vi "RSZVB Write From File To Instrument.vi"(8 "error in (no error)":errorcluster {"code" format="%.0x"}, 9 "Destination":path=path "D:/user/data/test.hcp", 10 "Source":path=path "C:/test.hcp", 11 "VISA session":refnum<visa-resource-name>) -> (0 "error out":errorcluster {"code" format="%.0x"}, 3 "dup VISA session":refnum<visa-resource-name>)   [LabVIEW 2011]
doc: "This VI is used to read data from the host computer and write it to a user specified file in the instrument.\n\nRemote-control command(s):\nSYSTem:COMMunicate:GPIB[:SELF]:RTERminator LFEOI | EOI\nMMEMory:DATA '<file_name>', <data>"
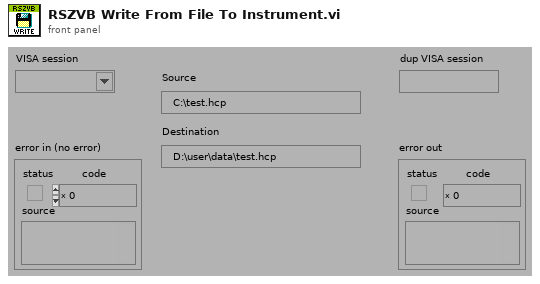
[diagram p1: front panel]
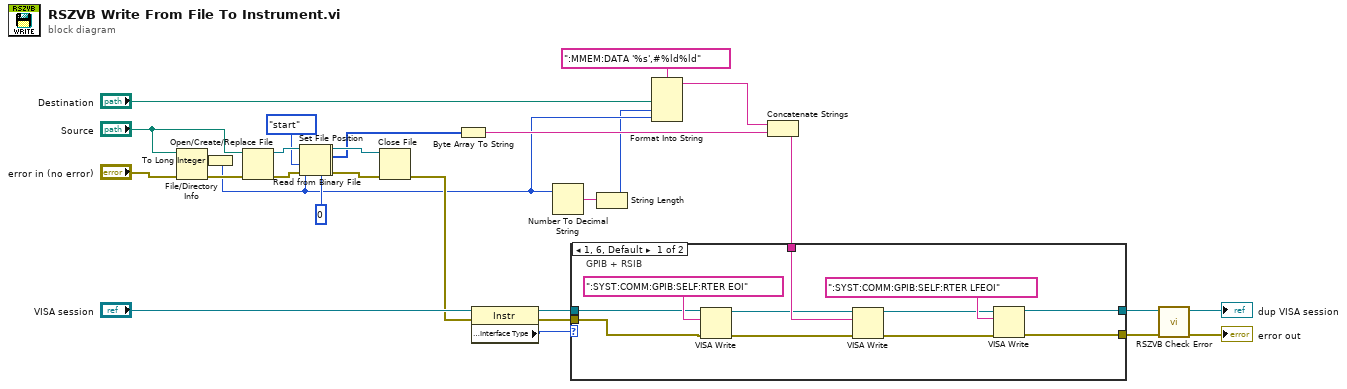
[diagram p0: block diagram]
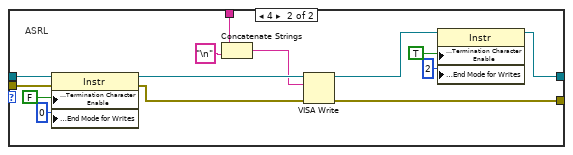
[diagram p2: hidden frame]
diagram:
  n1 = File/Directory Info(path="Source", error in="error in (no error)") -> (size=w3:i64, error out=w19:errorcluster)  [unwired: 5 out]
  n2 = To Long Integer(number=w3) -> (32bit integer=w9:i32)
  n3 = Open/Create/Replace File(file path (use dialog)="Source", error in=w19) -> (refnum out=w17:refnum<file>, error out=w21:errorcluster)  [unwired: 4 in, 1 out]
  n4 = Set File Position(refnum=w17, from (0:start)=enum16{"start", "end", "current"}."start" ("pos mode (0:2)"), error in=w21) -> (refnum out=w2:refnum<file>, error out=w1:errorcluster)  [unwired: 1 in]
  n5 = Read from Binary File(5:u8 0 ("byte stream type"), 8:w1, 10:w9, 11:w2) -> (0:w20:errorcluster, 2:w13:u8[], 3:w18:refnum<file>)  [unwired: 2 in, 1 out]
  n6 = Close File(refnum=w18, error in=w20) -> (error out=w11:errorcluster)  [unwired: 1 out]
  n7 = Byte Array To String(unsigned byte array=w13) -> (string=w12:string)
  n8 = property class="Instr"(reference="VISA session", error in=w11) -> (reference out=w27:refnum<visa-resource-name>, error out=w26:errorcluster, "Interface Information:Interface Type"=w25:u16)
  n9 = Number To Decimal String(number=w9) -> (decimal integer string=w10:string)  [unwired: 1 in]
  n10 = String Length(string=w10) -> (length=w8:i32)
  n11 = Format Into String(format string=":MMEM:DATA '%s',#%ld%ld", "Destination", w8, w9) -> (resulting string=w30:string)  [unwired: 2 in, 1 out]
  n12 = Concatenate Strings(w30, w12) -> (w28:string)
  n13 = case shown="1, 6, Default" w25 {
    tunnel: [w41 w45] -> w4
    tunnel: [w40 w44] -> w5
    tunnel: w28 -> [w39 w49]
    tunnel: w27 -> [w32 w55]
    tunnel: w26 -> [w31 w54]
    frame 1, 6, Default {
      # "GPIB + RSIB"
      n14 = VISA Write(VISA resource name=w32, write buffer=":SYST:COMM:GPIB:SELF:RTER EOI", error in (no error)=w31) -> (VISA resource name out=w36:refnum<visa-resource-name>, error out=w33:errorcluster)  [unwired: 1 out]
      n15 = VISA Write(VISA resource name=w36, write buffer=w39, error in (no error)=w33) -> (VISA resource name out=w35:refnum<visa-resource-name>, error out=w34:errorcluster)  [unwired: 1 out]
      n16 = VISA Write(VISA resource name=w35, write buffer=":SYST:COMM:GPIB:SELF:RTER LFEOI", error in (no error)=w34) -> (VISA resource name out=w40:refnum<visa-resource-name>, error out=w41:errorcluster)  [unwired: 1 out]
    }
    frame 4 {
      # "ASRL"
      n17 = property class="Instr"(reference=w55, error in=w54, "Message Based Settings:Termination Character Enable"=FALSE ("TermChar En"), "Serial Settings:End Mode for Writes"=u16 0 ("ASRL End Out")) -> (reference out=w51:refnum<visa-resource-name>, error out=w50:errorcluster)
      n18 = Concatenate Strings(w49, "\n") -> (w47:string)
      n19 = VISA Write(VISA resource name=w51, write buffer=w47, error in (no error)=w50) -> (VISA resource name out=w46:refnum<visa-resource-name>, error out=w45:errorcluster)  [unwired: 1 out]
      n20 = property class="Instr"(reference=w46, "Message Based Settings:Termination Character Enable"=TRUE ("TermChar En"), "Serial Settings:End Mode for Writes"=u16 2 ("ASRL End Out")) -> (reference out=w44:refnum<visa-resource-name>)  [unwired: 1 in, 1 out]
    }
  }
  n21 = call "RSZVB Check Error.vi"("error in (no error)"=w4, "VISA session"=w5) -> ("error out"=→"error out":errorcluster, "dup VISA session"=→"dup VISA session":refnum<visa-resource-name>)  [unwired: 8 in]
